vi "empty_point_array_2d.vi"() -> (0 "Array":cluster{"X":i32, "Y":i32}[][](array[cluster]))   [LabVIEW 2017]
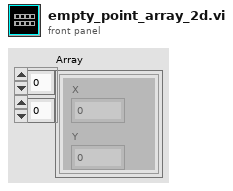
[diagram p1: front panel]
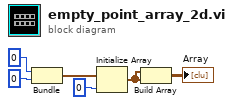
[diagram p0: block diagram]
diagram:
  n1 = Bundle(0, 0) -> (w6:cluster{i32, i32})  [unwired: 1 in]
  n2 = Initialize Array(w6, 0 ("dimension size")) -> (w1:cluster{i32, i32}[])
  n3 = Build Array(w1, w1) -> (→"Array":cluster{i32, i32}[][])
